vi "Add Test Event To Tree.vi"(8 "error in (no error)":errorcluster, 9 "Test Event":T1={"Name"="", "Passed"=FALSE, "Call Chain"=[], "Test Error"={"status"=FALSE, "code"=0, "source"=""}, "Time Stamp"=timestamp(0 s since 1904-01-01), "Unique Assert ID"="", "Test ID"="", "Execution time (s)"=-1.0, "Verbose Explanation"=""}, 10 "Parent Key":string, 11 "tree refnum":refnum<vi>) -> (0 "error out":errorcluster, 3 "dup tree refnum":refnum<vi>)   [LabVIEW 2013, in "Caraya.lvlib" / "Basic Test Manager.lvclass"]
uses:
  Basic Test Manager.lvclass
  Test Result/Assert Event Data.ctl
  Test Result/Test Result.lvclass
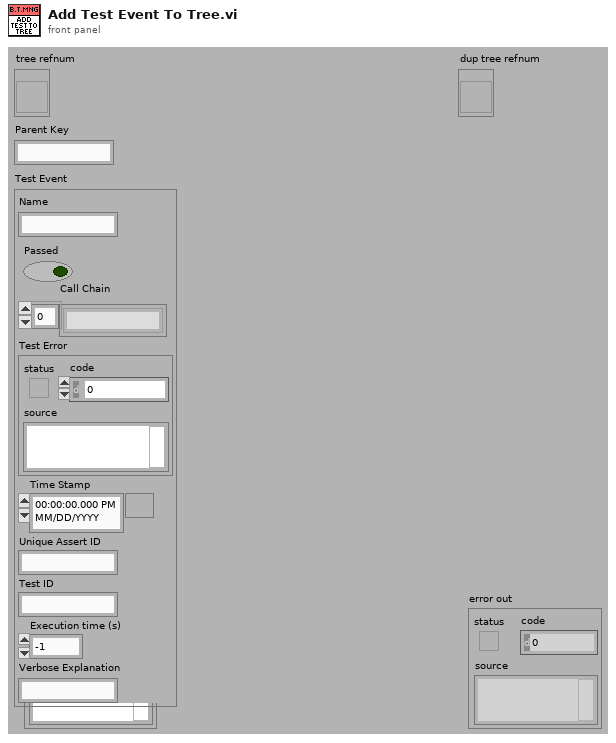
[diagram p1: front panel]
types:
  T1 = typedef "Caraya.lvlib/Test Result.lvclass/Assert Event Data.ctl" = cluster{"Name":string, "Passed":bool, "Call Chain":string[], "Test Error":errorcluster, "Time Stamp":timestamp, "Unique Assert ID":string, "Test ID":string, "Execution time (s)":dbl, "Verbose Explanation":string}
  T2 = typedef "Caraya.lvlib/Basic Test Manager.lvclass/Test State.ctl" = enum16{"Empty", "Unknown", "Fail", "Pass", "Skip", "Error"}
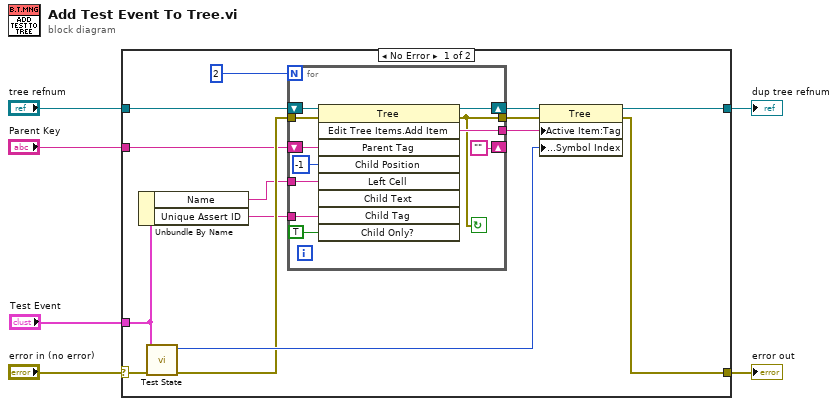
[diagram p0: block diagram]
diagram:
  n1 = case shown="No Error" "error in (no error)" {
    selector: "error in (no error)" -> [w11 w33]
    tunnel: [w14 w33] -> w5
    tunnel: [w18 w32] -> w3
    tunnel: "tree refnum" -> [w20 w32]
    tunnel: "Parent Key" -> [w9 _]
    tunnel: "Test Event" -> [w12 _]
    frame No Error {
      n2 = Unbundle By Name(w12) -> ("Name"=w8:string, "Unique Assert ID"=w7:string)
      n3 = call "Test State.vi"("error in (no error)"=w11, "Test Event"=w12) -> ("error out"=w10:errorcluster, "Test State"=w16:T2)  [unwired: 8 in]
      n4 = for {
        N: 2 -> [_]
        tunnel: w8 -> [w27]
        tunnel: [w26] -> w17
        shift-right: [w28] -> w19
        shift-left: w20 -> [w31]
        tunnel: w10 -> [w25]
        tunnel: [w24] -> w15
        shift-right: [""] -> _
        shift-left: w9 -> [w30]
        tunnel: w7 -> [w21]
        stop <- w24 continue-if-true
        n5 = invoke on="Invoke Node" class="Tree" method="Edit Tree Items.Add Item"(reference=w31, error in=w25, "Parent Tag"=w30, "Child Position"=-1, "Left Cell"=w27, "Child Tag"=w21, "Child Only?"=TRUE) -> (reference out=w28:refnum<vi>, error out=w24:errorcluster, "Edit Tree Items:Add Item"=w26:string)  [unwired: 2 in, 6 out]
      }
      n6 = property class="Tree"(reference=w19, error in=w15, "Active Item:Tag"=w17, "Active Item:Symbol Index"=w16) -> (reference out=w18:refnum<vi>, error out=w14:errorcluster)
    }
    frame Error {
    }
  }
  "error out" <- w5
  "dup tree refnum" <- w3
